vi "Get Status Channel.vi"(8 "error in":errorcluster, 11 "section reference in":T1 format="%.0x") -> (0 "error out":errorcluster, 2 "status channel":T1 format="%.0x", 3 "section reference out":T1 format="%.0x", 4 "found?":bool)   [LabVIEW 2020, in "Ballard MIL-STD-1553 Scripting.lvlib"]
uses:
  Ballard MIL-STD-1553 Scripting.lvlib
  <vilib>/NI VeriStand/Custom Device API/Custom Device Item Ref.ctl
  Constants.vi
  <vilib>/NI VeriStand/Custom Device Tools/Custom Device Utility Library/NI VeriStand - Search for Item by GUID.vi
  <vilib>/NI VeriStand/Custom Device Tools/Custom Device Utility Library/Custom Device Utility Library.lvlib
  <vilib>/NI VeriStand/Custom Device API/Custom Device API.lvlib
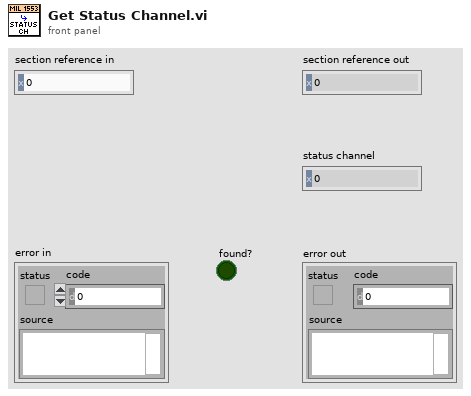
[diagram p1: front panel]
types:
  T1 = typedef "Custom Device API.lvlib/Custom Device Item Ref.ctl" = u64
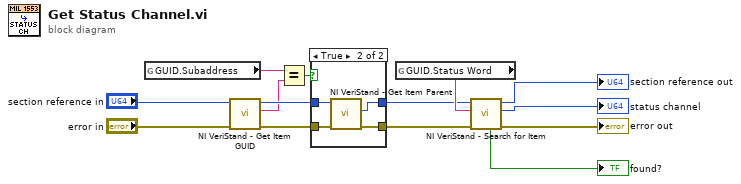
[diagram p0: block diagram]
diagram:
  n1 = global read "Constants.vi" "GUID.Subaddress"() -> (w5:string)
  n2 = call <vilib>:"NI VeriStand - Get Item GUID.vi"("error in (no error)"="error in", "Item Ref in"="section reference in") -> ("error out"=w8:errorcluster, "GUID"=w6:string, "Item Ref out"=w9:T1)  [unwired: 7 in]
  n3 = Equal?(x=w5, y=w6) -> (x = y?=w7:bool)
  n4 = case shown="True" w7 {
    tunnel: w9 -> [w16 w20]
    tunnel: w8 -> [w15 w19]
    tunnel: [w16 w17] -> w1
    tunnel: [w15 w18] -> w2
    frame False {
    }
    frame True {
      n5 = call <vilib>:"NI VeriStand - Get Item Parent.vi"("error in (no error)"=w19, "Item Ref in"=w20) -> ("error out"=w18:errorcluster, "Parent Ref"=w17:T1)  [unwired: 6 in, 2 out]
    }
  }
  n6 = global read "Constants.vi" "GUID.Status Word"() -> (w13:string)
  n7 = call-poly <vilib>:"NI VeriStand - Search for Item.vi"("error in"=w2, "Item GUID"=w13, "Section Ref in"=w1) -> ("error out"=→"error out":errorcluster, "Item Ref"=→"status channel":T1, "Section Ref out"=→"section reference out":T1, "Found"=→"found?":bool)  [unwired: 5 in]
